vi "Parse Protocol.vi"(8 "error in (no error)":errorcluster, 11 "Protocol Cluster":variant) -> (0 "error out":errorcluster, 3 "Params Values":T1(array[cluster]))   [LabVIEW 2022 SP3, in "EClib functions.lvlib"]
doc: "This intermediate VI transform a cluster of parameters to an array. This transformation is realised by XML Functions."
uses:
  EClib functions.lvlib
  <vilib>/Utility/error.llb/Trim Whitespace One-Sided.vi
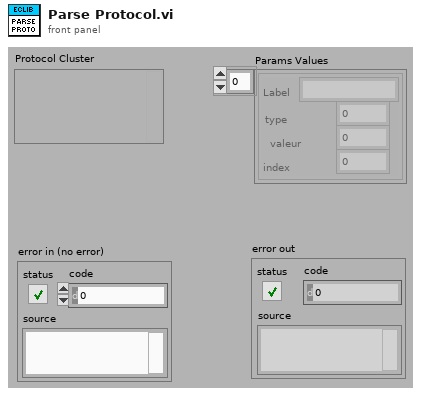
[diagram p1: front panel]
types:
  T1 = cluster{"Label":string, "type":i32, "valeur":u32, "index":i32}[]
  T2 = cluster{"string before end tag":string, i32, i32, i32}[]
  T3 = cluster{"trimmed string":string, i32, u32, i32}[]
  T4 = cluster{"trimmed string":string, i32, i32, i32}[]
  T5 = cluster{"Label":string, "type":i32, "valeur":u32, "index":i32}
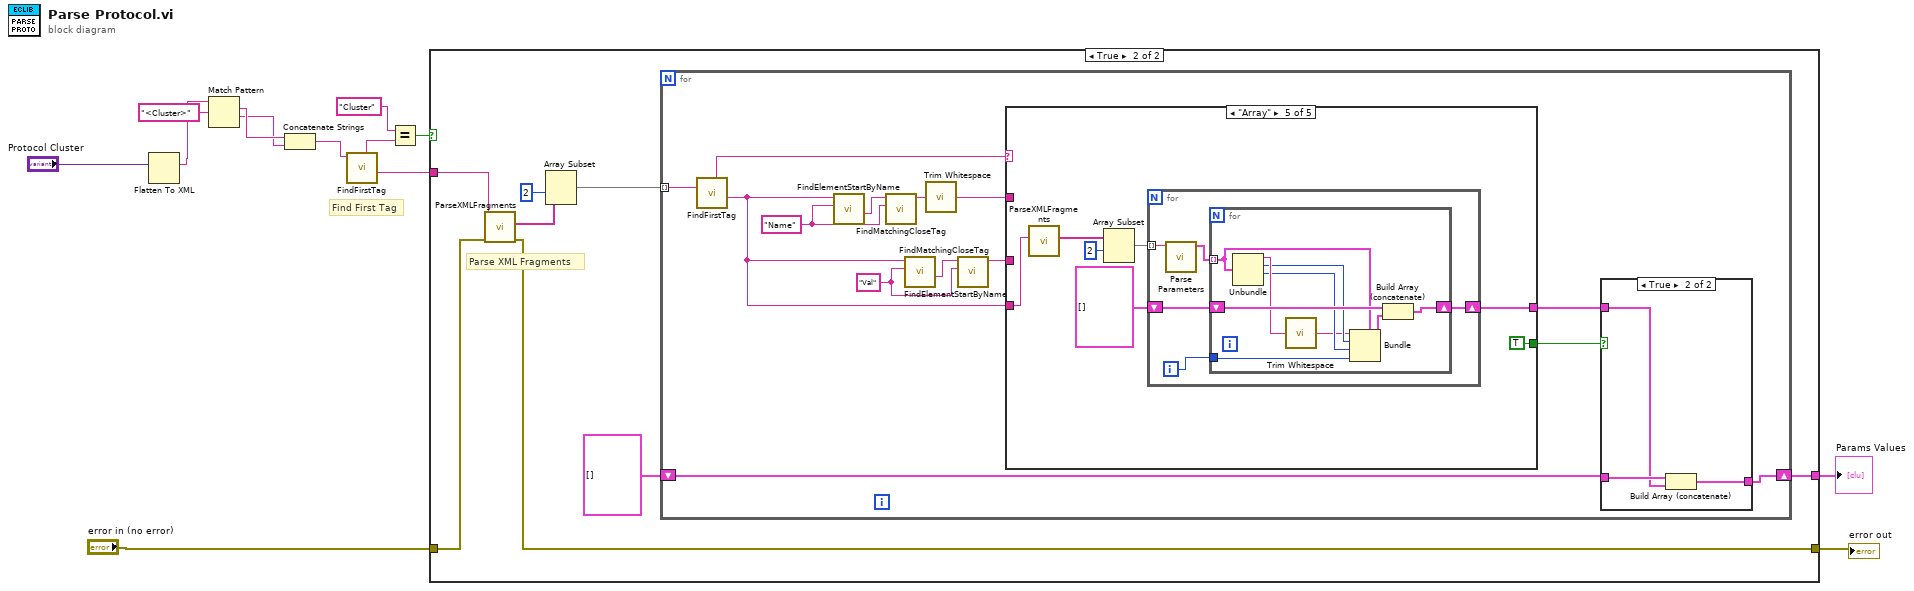
[diagram p0: block diagram]
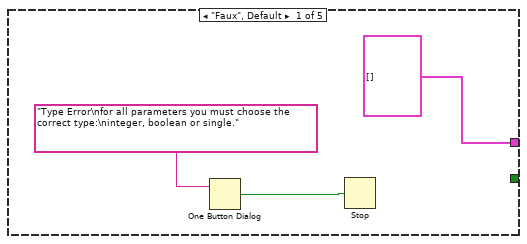
[diagram p4: hidden frame]
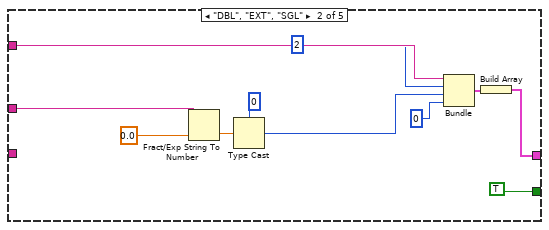
[diagram p5: hidden frame]
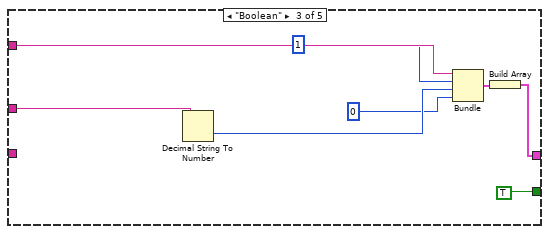
[diagram p6: hidden frame]
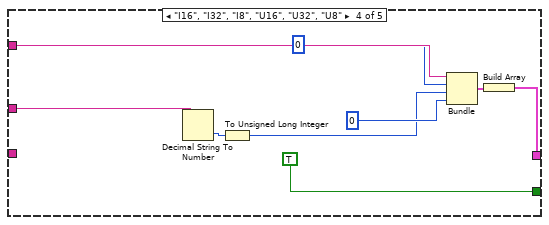
[diagram p7: hidden frame]
diagram:
  # "Find First Tag"
  n1 = Flatten To XML(6:"Protocol Cluster") -> (2:w5:string)
  n2 = Match Pattern(string=w5, regular expression="<Cluster>") -> (match substring=w3:string, after substring=w2:string)  [unwired: 1 in, 2 out]
  n3 = Concatenate Strings(w3, w2) -> (w1:string)
  n4 = call <vilib>:"FindFirstTag.vi"("XML String In"=w1) -> ("after tag"=w12:string, "element name"=w8:string)  [unwired: 5 in, 4 out]
  n5 = Equal?(x="Cluster" ("y"), y=w8) -> (x = y?=w13:bool)
  n6 = case shown="True" w13 {
    tunnel: w12 -> [_ w22]
    tunnel: [_ w18] -> w11
    tunnel: "error in (no error)" -> [w14 w16]
    tunnel: [w14 w15] -> w6
    frame False {
    }
    frame True {
      # "Parse XML Fragments"
      n7 = call <vilib>:"ParseXMLFragments.vi"("error in (no error)"=w16, "XML in"=w22) -> ("error out"=w15:errorcluster, "XML Elements"=w21:string[])  [unwired: 8 in]
      n8 = Array Subset(array=w21, index=2 ("indice")) -> (w19:string[])  [unwired: 1 in]
      n9 = for {
        tunnel: w19 -> [w36] mode=indexing
        shift-right: [w27] -> w18
        shift-left: T2 [] -> [w26]
        w30 = "Val" ("Element Name")
        w34 = "Name" ("Element Name")
        n10 = call <vilib>:"FindFirstTag.vi"("XML String In"=w36) -> ("after tag"=w28:string, "element name"=w35:string)  [unwired: 5 in, 4 out]
        n11 = call <vilib>:"FindElementStartByName.vi"("Element Name"=w34, "string"=w28) -> ("after substring"=w33:string)  [unwired: 6 in, 3 out]
        n12 = call <vilib>:"FindMatchingCloseTag.vi"("element name"=w34, "XML string in"=w33) -> ("string before end tag"=w32:string)  [unwired: 5 in, 4 out]
        n13 = call <vilib>:"FindElementStartByName.vi"("Element Name"=w30, "string"=w28) -> ("after substring"=w31:string)  [unwired: 6 in, 3 out]
        n14 = call <vilib>:"Trim Whitespace.vi"("string"=w32) -> ("trimmed string"=w24:string)  [unwired: 1 in]
        n15 = call <vilib>:"FindMatchingCloseTag.vi"("element name"=w30, "XML string in"=w31) -> ("string before end tag"=w29:string)  [unwired: 5 in, 4 out]
        n16 = case shown="\"Array\"" w35 {
          tunnel: w29 -> [_ w54 w61 w70 _]
          tunnel: w24 -> [_ w48 w59 w68 _]
          tunnel: [_ TRUE TRUE TRUE TRUE] -> w23
          tunnel: w28 -> [_ _ _ _ w75]
          tunnel: [T2 [] w45 w56 w65 w72] -> w25
          frame "Faux", Default {
            n17 = One Button Dialog(message="Type Error\nfor all parameters you must choose the correct type:\ninteger, boolean or single.") -> (true=w42:bool)  [unwired: 1 in]
            n18 = Stop(stop? (T)=w42) -> ()
          }
          frame "DBL", "EXT", "SGL" {
            n19 = Fract/Exp String To Number(string=w54, default (0 dbl)=sgl 0.0 ("valeur par défaut (0 DBL)")) -> (number=w52:sgl)  [unwired: 2 in, 1 out]
            n20 = Type Cast(type=u32 0, x=w52) -> (*(type *) &x=w46:u32)
            n21 = Bundle("trimmed string"=w48, 2, w46, 0) -> (w49:cluster{"trimmed string":string, i32, u32, i32})  [unwired: 1 in]
            n22 = Build Array(w49) -> (w45:T3)
          }
          frame "Boolean" {
            n23 = Decimal String To Number(string=w61) -> (number=w57:i32)  [unwired: 2 in, 1 out]
            n24 = Bundle("trimmed string"=w59, 1, w57, 0) -> (w60:cluster{"trimmed string":string, i32, i32, i32})  [unwired: 1 in]
            n25 = Build Array(w60) -> (w56:T4)
          }
          frame "I16", "I32", "I8", "U16", "U32", "U8" {
            n26 = Decimal String To Number(string=w70) -> (number=w66:i32)  [unwired: 2 in, 1 out]
            n27 = To Unsigned Long Integer(number=w66) -> (unsigned 32bit integer=w63:u32)
            n28 = Bundle("trimmed string"=w68, 0, w63, 0) -> (w69:cluster{"trimmed string":string, i32, u32, i32})  [unwired: 1 in]
            n29 = Build Array(w69) -> (w65:T3)
          }
          frame "Array" {
            n30 = call <vilib>:"ParseXMLFragments.vi"("XML in"=w75) -> ("XML Elements"=w78:string[])  [unwired: 9 in, 1 out]
            n31 = Array Subset(array=w78, index=2 ("indice")) -> (w76:string[])  [unwired: 1 in]
            n32 = for {
              tunnel: w76 -> [w80] mode=indexing
              shift-right: [w81] -> w72
              shift-left: T2 [] -> [w83]
              i -> [w82]
              n33 = call "Parse Parameters.vi"("XML String In"=w80) -> ("Params Values"=w79:T1)  [unwired: 7 in, 1 out]
              n34 = for {
                tunnel: w79 -> [w86] mode=indexing
                tunnel: w82 -> [w88]
                shift-right: [w85] -> w81
                shift-left: w83 -> [w92]
                n35 = Unbundle(w86) -> ("Label"=w91:string, "type"=w90:i32, "valeur"=w89:u32)  [unwired: 1 out]
                n36 = call <vilib>:"Trim Whitespace.vi"("string"=w91) -> ("trimmed string"=w84:string)  [unwired: 1 in]
                n37 = Bundle(cluster=w86, "Label"=w84, "type"=w90, "valeur"=w89, "index"=w88) -> (w87:T5)
                n38 = Build Array (concatenate)(w92, w87) -> (w85:T1)
              }
            }
          }
        }
        n39 = case shown="True" w23 {
          tunnel: w26 -> [w37 w40]
          tunnel: w25 -> [_ w39]
          tunnel: [w37 w38] -> w27
          frame False {
          }
          frame True {
            n40 = Build Array (concatenate)(w40, w39) -> (w38:T1)
          }
        }
      }
    }
  }
  "Params Values" <- w11
  "error out" <- w6
